vi "ActionVIOnLoad.vi"(8 "error in (no error)":errorcluster, 11 "Device Item Ref in":T1 format="%.0x") -> (0 "error out":errorcluster, 3 "Device Item Ref out":T1 format="%.0x")   [LabVIEW 2015, in "Chassis TimeSync System Explorer.lvlib"]
uses:
  Chassis TimeSync System Explorer.lvlib
  <vilib>/NI Veristand/Custom Device API/Custom Device Item Ref.ctl
  <vilib>/NI Veristand/Custom Device API/Custom Device API.lvlib
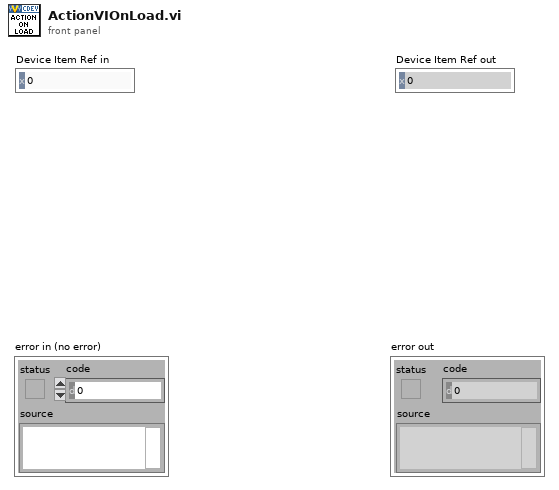
[diagram p1: front panel]
types:
  T1 = typedef "Custom Device API.lvlib/Custom Device Item Ref.ctl" = u64
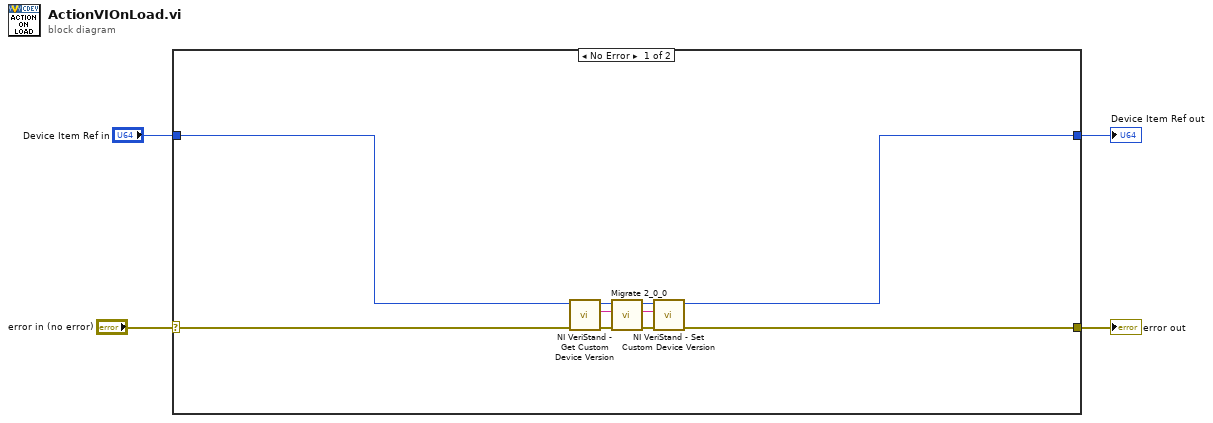
[diagram p0: block diagram]
diagram:
  n1 = case shown="No Error" "error in (no error)" {
    selector: "error in (no error)" -> [w13 w16]
    tunnel: [w6 w16] -> w3
    tunnel: "Device Item Ref in" -> [w14 w15]
    tunnel: [w5 w15] -> w1
    frame No Error {
      n2 = call <vilib>:"NI VeriStand - Get Custom Device Version.vi"("error in (no error)"=w13, "Device Ref in"=w14) -> ("error out"=w11:errorcluster, "Value"=w10:string, "Device Ref out"=w12:T1)  [unwired: 7 in]
      n3 = call "Migrate 2_0_0.vi"("error in (no error)"=w11, "version"=w10, "Device Ref in"=w12) -> ("error out"=w7:errorcluster, "new version"=w8:string, "Device Ref out"=w9:T1)  [unwired: 6 in]
      n4 = call <vilib>:"NI VeriStand - Set Custom Device Version.vi"("error in (no error)"=w7, "Value"=w8, "Device Ref in"=w9) -> ("error out"=w6:errorcluster, "Device Ref out"=w5:T1)  [unwired: 7 in]
    }
    frame Error {
    }
  }
  "error out" <- w3
  "Device Item Ref out" <- w1
